vi "WriteGeneralData.vi"(0 "filename (discard if empty)":string, 1 "Array":dbl[][](array[numeric]), 2 "Column name array":string[](array[string])) -> ()   [LabVIEW 2017]
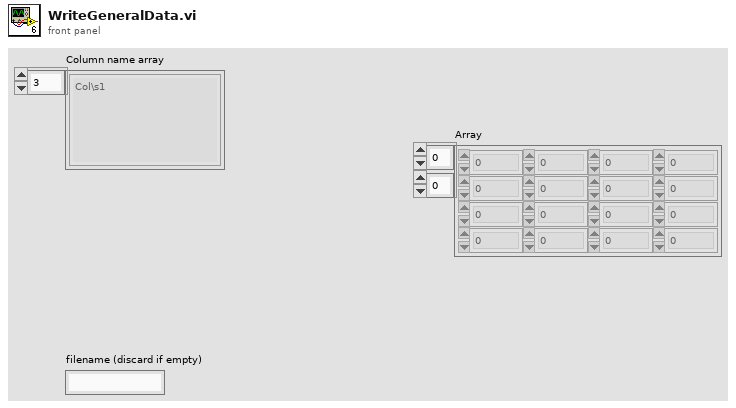
[diagram p1: front panel]
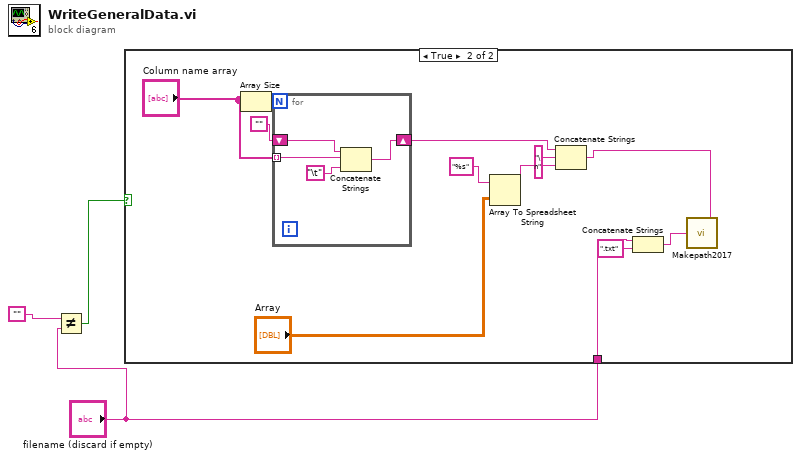
[diagram p0: block diagram]
diagram:
  n1 = Not Equal?(x="", y="filename (discard if empty)") -> (x != y?=w1:bool)
  n2 = case shown="True" w1 {
    tunnel: "filename (discard if empty)" -> [_ w10]
    frame False {
    }
    frame True {
      n3 = Array Size(array="Column name array") -> (size(s)=w7:i32)
      n4 = for {
        N: w7 -> [_]
        tunnel: "Column name array" -> [w19] mode=indexing
        shift-right: [w17] -> w4
        shift-left: "" -> [w18]
        n5 = Concatenate Strings(w18, w19, "\t") -> (w17:string)
      }
      n6 = Array To Spreadsheet String(array="Array", 3:"%s" ("format string")) -> (spreadsheet string=w15:string)  [unwired: 1 in]
      n7 = Concatenate Strings(w4, "\n" ("string"), w15) -> (w14:string)
      n8 = Concatenate Strings(w10, ".txt" ("string")) -> (w11:string)
      n9 = call "Makepath2017.vi"("text to save"=w14, "File name, format \\filename"=w11) -> ()
    }
  }
